vi "HEWH Flow Temp Adjust.vi"(0 "Core HEWH Data in":T5={"Scan Rate Adjust"=0.0, "Draw Count"=0, "Test Patten Setup"={"Total Gallons Schedule"=[], "PRAT/RLT Sequence"=[{"Sequence #"=1.0, "Cycles"=35, "Mode Setting"="", "Flow Rate (GPM)"=0.0, "Temperature (F)"=0.0, "Reset Timer"=FALSE, "Use Temp Decline Method"=FALSE, "Terminate Condition"=enum."C1-Terminate Draw @ Gallon Mark", "Condition Value #1"=0.0, "UE"=FALSE, "LE"=FALSE, "Comp"=FALSE, "Fan"=FALSE, "Test End Time (Sec)"=0.0, "Purge Until Cutout"=FALSE, "Start Conditions"=enum."Heat Source Cutout", "Condition Value #2"=0.0, "Remove Power"=FALSE, "Time"=0.0, "Check Special Cond."=enum."SC1-Do Nothing", "Condition#"=enum."C1", "Draw Flags"=enum."N/A", "Data Processing Delay (FHD 15sec, UEF 5 Sec)"=0.0, "Test Complete"=FALSE}, {"Sequence #"=2.0, "Cycles"=15, "Mode Setting"="", "Flow Rate (GPM)"=0.0, "Temperature (F)"=0.0, "Reset Timer"=FALSE, "Use Temp Decline Method"=FALSE, "Terminate Condition"=enum."C1-Terminate Draw @ Gallon Mark", "Condition Value #1"=0.0, "UE"=FALSE, "LE"=FALSE, "Comp"=FALSE, "Fan"=FALSE, "Test End Time (Sec)"=0.0, "Purge Until Cutout"=FALSE, "Start Conditions"=enum."Heat Source Cutout", "Condition Value #2"=0.0, "Remove Power"=FALSE, "Time"=0.0, "Check Special Cond."=enum."SC1-Do Nothing", "Condition#"=enum."C1", "Draw Flags"=enum."N/A", "Data Processing Delay (FHD 15sec, UEF 5 Sec)"=0.0, "Test Complete"=FALSE}, {"Sequence #"=3.0, "Cycles"=35, "Mode Setting"="", "Flow Rate (GPM)"=0.0, "Temperature (F)"=0.0, "Reset Timer"=FALSE, "Use Temp Decline Method"=FALSE, "Terminate Condition"=enum."C1-Terminate Draw @ Gallon Mark", "Condition Value #1"=0.0, "UE"=FALSE, "LE"=FALSE, "Comp"=FALSE, "Fan"=FALSE, "Test End Time (Sec)"=0.0, "Purge Until Cutout"=FALSE, "Start Conditions"=enum."Heat Source Cutout", "Condition Value #2"=0.0, "Remove Power"=FALSE, "Time"=0.0, "Check Special Cond."=enum."SC1-Do Nothing", "Condition#"=enum."C1", "Draw Flags"=enum."N/A", "Data Processing Delay (FHD 15sec, UEF 5 Sec)"=0.0, "Test Complete"=FALSE}, {"Sequence #"=4.0, "Cycles"=15, "Mode Setting"="", "Flow Rate (GPM)"=0.0, "Temperature (F)"=0.0, "Reset Timer"=FALSE, "Use Temp Decline Method"=FALSE, "Terminate Condition"=enum."C1-Terminate Draw @ Gallon Mark", "Condition Value #1"=0.0, "UE"=FALSE, "LE"=FALSE, "Comp"=FALSE, "Fan"=FALSE, "Test End Time (Sec)"=0.0, "Purge Until Cutout"=FALSE, "Start Conditions"=enum."Heat Source Cutout", "Condition Value #2"=0.0, "Remove Power"=FALSE, "Time"=0.0, "Check Special Cond."=enum."SC1-Do Nothing", "Condition#"=enum."C1", "Draw Flags"=enum."N/A", "Data Processing Delay (FHD 15sec, UEF 5 Sec)"=0.0, "Test Complete"=FALSE}, {"Sequence #"=5.0, "Cycles"=35, "Mode Setting"="", "Flow Rate (GPM)"=0.0, "Temperature (F)"=0.0, "Reset Timer"=FALSE, "Use Temp Decline Method"=FALSE, "Terminate Condition"=enum."C1-Terminate Draw @ Gallon Mark", "Condition Value #1"=0.0, "UE"=FALSE, "LE"=FALSE, "Comp"=FALSE, "Fan"=FALSE, "Test End Time (Sec)"=0.0, "Purge Until Cutout"=FALSE, "Start Conditions"=enum."Heat Source Cutout", "Condition Value #2"=0.0, "Remove Power"=FALSE, "Time"=0.0, "Check Special Cond."=enum."SC1-Do Nothing", "Condition#"=enum."C1", "Draw Flags"=enum."N/A", "Data Processing Delay (FHD 15sec, UEF 5 Sec)"=0.0, "Test Complete"=FALSE}, {"Sequence #"=6.0, "Cycles"=15, "Mode Setting"="", "Flow Rate (GPM)"=0.0, "Temperature (F)"=0.0, "Reset Timer"=FALSE, "Use Temp Decline Method"=FALSE, "Terminate Condition"=enum."C1-Terminate Draw @ Gallon Mark", "Condition Value #1"=0.0, "UE"=FALSE, "LE"=FALSE, "Comp"=FALSE, "Fan"=FALSE, "Test End Time (Sec)"=0.0, "Purge Until Cutout"=FALSE, "Start Conditions"=enum."Heat Source Cutout", "Condition Value #2"=0.0, "Remove Power"=FALSE, "Time"=0.0, "Check Special Cond."=enum."SC1-Do Nothing", "Condition#"=enum."C1", "Draw Flags"=enum."N/A", "Data Processing Delay (FHD 15sec, UEF 5 Sec)"=0.0, "Test Complete"=FALSE}, {"Sequence #"=7.0, "Cycles"=35, "Mode Setting"="", "Flow Rate (GPM)"=0.0, "Temperature (F)"=0.0, "Reset Timer"=FALSE, "Use Temp Decline Method"=FALSE, "Terminate Condition"=enum."C1-Terminate Draw @ Gallon Mark", "Condition Value #1"=0.0, "UE"=FALSE, "LE"=FALSE, "Comp"=FALSE, "Fan"=FALSE, "Test End Time (Sec)"=0.0, "Purge Until Cutout"=FALSE, "Start Conditions"=enum."Heat Source Cutout", "Condition Value #2"=0.0, "Remove Power"=FALSE, "Time"=0.0, "Check Special Cond."=enum."SC1-Do Nothing", "Condition#"=enum."C1", "Draw Flags"=enum."N/A", "Data Processing Delay (FHD 15sec, UEF 5 Sec)"=0.0, "Test Complete"=FALSE}, {"Sequence #"=8.0, "Cycles"=15, "Mode Setting"="", "Flow Rate (GPM)"=0.0, "Temperature (F)"=0.0, "Reset Timer"=FALSE, "Use Temp Decline Method"=FALSE, "Terminate Condition"=enum."C1-Terminate Draw @ Gallon Mark", "Condition Value #1"=0.0, "UE"=FALSE, "LE"=FALSE, "Comp"=FALSE, "Fan"=FALSE, "Test End Time (Sec)"=0.0, "Purge Until Cutout"=FALSE, "Start Conditions"=enum."Heat Source Cutout", "Condition Value #2"=0.0, "Remove Power"=FALSE, "Time"=0.0, "Check Special Cond."=enum."SC1-Do Nothing", "Condition#"=enum."C1", "Draw Flags"=enum."N/A", "Data Processing Delay (FHD 15sec, UEF 5 Sec)"=0.0, "Test Complete"=FALSE}], "Current Sequence Index"=0}, "HEWH Specific DAQ"={"HEWH Data"={"HEWH Standard"={"Voltage (Volts)"=0.0, "Current (Amps)"=0.0, "Power (Watts)"=0.0, "WattHours (Wh)"=0.0, "TC Tree (AVG)"=0.0, "Flow Rate (GPM)"=0.0, "Gallons (Gal)"=0.0, "RTD Out (Deg F)"=0.0, "RTD In (Deg F)"=0.0, "RTD Amb (Deg F)"=0.0, "TC Down"=0.0, "UE Event Lead"=0, "LE Event Lead"=0, "TC Tree Array"=[]}, "PRAT"={"Power (Watts) A"=4192.0, "Power (Watts) B"=4192.0, "Power (Watts) C"=4192.0, "Power (Watts) D"=4192.0, "TC1"=0.0, "TC2"=0.0, "TC3"=0.0, "TC4"=0.0, "WattHours (Wh) A"=4192.0, "WattHours (Wh) B"=4192.0, "WattHours (Wh) C"=4192.0, "WattHours (Wh) D"=4192.0, "Ambient"=0.0, "Extra Temp"=0.0}, "Additional Power Data"={"Vthd"=236.2, "Frequency (Hz)"=236.2, "Apparent Power (VA)"=236.2, "Power Factor"=236.2, "Current Crest Factor"=236.2, "Voltage Crest Factor"=236.2, "Integration Time (sec)"=236.2}}, "Flow Valve % Open"=0.0, "Power State"={"UE"=FALSE, "LE"=FALSE, "COMP"=FALSE, "FANS"=FALSE}, "Power Analyzer"=enum."", "Flow Valve uA Output"=0, "Gallons Start (Gal)"=0.0}, "Test Output Data"={"PreDraw Data Table"=[], "Data Table"=[], "MW100 TC Headers"=[]}, "Calc and Calibration"={"Mean SD Var Max Min Array"=[], "Draw Statistics (DBL)"=[], "Calibration Coefficients DBL"=[], "Start Gallons"=0.0, "Starting Temp Decline"=0.0, "K-Factor (Intellifaucet)"=0.0, "All Draw Stats"=[], "RTD Terminate Value"=0.0}, "Current Draw Time"=0.0, "LV Program"=enum."HEWH", "Station ID"=enum."A", "Current Cond"=enum."N/A", "Test Complete"=FALSE} {"Test Patten Setup"."PRAT/RLT Sequence"."Time" format="%<%H:%M:%S>t"; "Test Patten Setup"."Total Gallons Schedule" format="%.2f"}, 1 "MW100":refnum<visa-resource-name>, 2 "Yokogawa WT210":refnum<visa-resource-name>, 3 "Temperature":T2 format="%.2f", 4 "Gallon Target":T2=10.72 format="%.2f", 5 "error in (no error)":errorcluster, 6 "Debug":bool, 7 "Purge Time (Seconds)":T2=180.0 format="%.2f", 8 "Use Fuzzy Logic":bool, 9 "PID gains (Temp)":T1={"proportional gain (Kc)"=0.1, "integral time (Ti, min)"=0.01, "derivative time (Td, min)"=0.0} {"derivative time (Td, min)" format="%.3f"; "integral time (Ti, min)" format="%.3f"; "proportional gain (Kc)" format="%.3f"}, 10 "GEA2?":bool, 11 "GPM Target":T2=3.0 format="%.2f", 12 "State":T4, 13 "MW100 Sema":T3, 16 "Use Emerson 5700?":bool, 17 "Pressurization Time (sec)":i32, 18 "Laurel IP Address":string) -> (14 "Core HEWH Data out":T5={"Scan Rate Adjust"=0.0, "Draw Count"=0, "Test Patten Setup"={"Total Gallons Schedule"=[], "PRAT/RLT Sequence"=[{"Sequence #"=1.0, "Cycles"=35, "Mode Setting"="", "Flow Rate (GPM)"=0.0, "Temperature (F)"=0.0, "Reset Timer"=FALSE, "Use Temp Decline Method"=FALSE, "Terminate Condition"=enum."C1-Terminate Draw @ Gallon Mark", "Condition Value #1"=0.0, "UE"=FALSE, "LE"=FALSE, "Comp"=FALSE, "Fan"=FALSE, "Test End Time (Sec)"=0.0, "Purge Until Cutout"=FALSE, "Start Conditions"=enum."Heat Source Cutout", "Condition Value #2"=0.0, "Remove Power"=FALSE, "Time"=0.0, "Check Special Cond."=enum."SC1-Do Nothing", "Condition#"=enum."C1", "Draw Flags"=enum."N/A", "Data Processing Delay (FHD 15sec, UEF 5 Sec)"=0.0, "Test Complete"=FALSE}, {"Sequence #"=2.0, "Cycles"=15, "Mode Setting"="", "Flow Rate (GPM)"=0.0, "Temperature (F)"=0.0, "Reset Timer"=FALSE, "Use Temp Decline Method"=FALSE, "Terminate Condition"=enum."C1-Terminate Draw @ Gallon Mark", "Condition Value #1"=0.0, "UE"=FALSE, "LE"=FALSE, "Comp"=FALSE, "Fan"=FALSE, "Test End Time (Sec)"=0.0, "Purge Until Cutout"=FALSE, "Start Conditions"=enum."Heat Source Cutout", "Condition Value #2"=0.0, "Remove Power"=FALSE, "Time"=0.0, "Check Special Cond."=enum."SC1-Do Nothing", "Condition#"=enum."C1", "Draw Flags"=enum."N/A", "Data Processing Delay (FHD 15sec, UEF 5 Sec)"=0.0, "Test Complete"=FALSE}, {"Sequence #"=3.0, "Cycles"=35, "Mode Setting"="", "Flow Rate (GPM)"=0.0, "Temperature (F)"=0.0, "Reset Timer"=FALSE, "Use Temp Decline Method"=FALSE, "Terminate Condition"=enum."C1-Terminate Draw @ Gallon Mark", "Condition Value #1"=0.0, "UE"=FALSE, "LE"=FALSE, "Comp"=FALSE, "Fan"=FALSE, "Test End Time (Sec)"=0.0, "Purge Until Cutout"=FALSE, "Start Conditions"=enum."Heat Source Cutout", "Condition Value #2"=0.0, "Remove Power"=FALSE, "Time"=0.0, "Check Special Cond."=enum."SC1-Do Nothing", "Condition#"=enum."C1", "Draw Flags"=enum."N/A", "Data Processing Delay (FHD 15sec, UEF 5 Sec)"=0.0, "Test Complete"=FALSE}, {"Sequence #"=4.0, "Cycles"=15, "Mode Setting"="", "Flow Rate (GPM)"=0.0, "Temperature (F)"=0.0, "Reset Timer"=FALSE, "Use Temp Decline Method"=FALSE, "Terminate Condition"=enum."C1-Terminate Draw @ Gallon Mark", "Condition Value #1"=0.0, "UE"=FALSE, "LE"=FALSE, "Comp"=FALSE, "Fan"=FALSE, "Test End Time (Sec)"=0.0, "Purge Until Cutout"=FALSE, "Start Conditions"=enum."Heat Source Cutout", "Condition Value #2"=0.0, "Remove Power"=FALSE, "Time"=0.0, "Check Special Cond."=enum."SC1-Do Nothing", "Condition#"=enum."C1", "Draw Flags"=enum."N/A", "Data Processing Delay (FHD 15sec, UEF 5 Sec)"=0.0, "Test Complete"=FALSE}, {"Sequence #"=5.0, "Cycles"=35, "Mode Setting"="", "Flow Rate (GPM)"=0.0, "Temperature (F)"=0.0, "Reset Timer"=FALSE, "Use Temp Decline Method"=FALSE, "Terminate Condition"=enum."C1-Terminate Draw @ Gallon Mark", "Condition Value #1"=0.0, "UE"=FALSE, "LE"=FALSE, "Comp"=FALSE, "Fan"=FALSE, "Test End Time (Sec)"=0.0, "Purge Until Cutout"=FALSE, "Start Conditions"=enum."Heat Source Cutout", "Condition Value #2"=0.0, "Remove Power"=FALSE, "Time"=0.0, "Check Special Cond."=enum."SC1-Do Nothing", "Condition#"=enum."C1", "Draw Flags"=enum."N/A", "Data Processing Delay (FHD 15sec, UEF 5 Sec)"=0.0, "Test Complete"=FALSE}, {"Sequence #"=6.0, "Cycles"=15, "Mode Setting"="", "Flow Rate (GPM)"=0.0, "Temperature (F)"=0.0, "Reset Timer"=FALSE, "Use Temp Decline Method"=FALSE, "Terminate Condition"=enum."C1-Terminate Draw @ Gallon Mark", "Condition Value #1"=0.0, "UE"=FALSE, "LE"=FALSE, "Comp"=FALSE, "Fan"=FALSE, "Test End Time (Sec)"=0.0, "Purge Until Cutout"=FALSE, "Start Conditions"=enum."Heat Source Cutout", "Condition Value #2"=0.0, "Remove Power"=FALSE, "Time"=0.0, "Check Special Cond."=enum."SC1-Do Nothing", "Condition#"=enum."C1", "Draw Flags"=enum."N/A", "Data Processing Delay (FHD 15sec, UEF 5 Sec)"=0.0, "Test Complete"=FALSE}, {"Sequence #"=7.0, "Cycles"=35, "Mode Setting"="", "Flow Rate (GPM)"=0.0, "Temperature (F)"=0.0, "Reset Timer"=FALSE, "Use Temp Decline Method"=FALSE, "Terminate Condition"=enum."C1-Terminate Draw @ Gallon Mark", "Condition Value #1"=0.0, "UE"=FALSE, "LE"=FALSE, "Comp"=FALSE, "Fan"=FALSE, "Test End Time (Sec)"=0.0, "Purge Until Cutout"=FALSE, "Start Conditions"=enum."Heat Source Cutout", "Condition Value #2"=0.0, "Remove Power"=FALSE, "Time"=0.0, "Check Special Cond."=enum."SC1-Do Nothing", "Condition#"=enum."C1", "Draw Flags"=enum."N/A", "Data Processing Delay (FHD 15sec, UEF 5 Sec)"=0.0, "Test Complete"=FALSE}, {"Sequence #"=8.0, "Cycles"=15, "Mode Setting"="", "Flow Rate (GPM)"=0.0, "Temperature (F)"=0.0, "Reset Timer"=FALSE, "Use Temp Decline Method"=FALSE, "Terminate Condition"=enum."C1-Terminate Draw @ Gallon Mark", "Condition Value #1"=0.0, "UE"=FALSE, "LE"=FALSE, "Comp"=FALSE, "Fan"=FALSE, "Test End Time (Sec)"=0.0, "Purge Until Cutout"=FALSE, "Start Conditions"=enum."Heat Source Cutout", "Condition Value #2"=0.0, "Remove Power"=FALSE, "Time"=0.0, "Check Special Cond."=enum."SC1-Do Nothing", "Condition#"=enum."C1", "Draw Flags"=enum."N/A", "Data Processing Delay (FHD 15sec, UEF 5 Sec)"=0.0, "Test Complete"=FALSE}], "Current Sequence Index"=0}, "HEWH Specific DAQ"={"HEWH Data"={"HEWH Standard"={"Voltage (Volts)"=0.0, "Current (Amps)"=0.0, "Power (Watts)"=0.0, "WattHours (Wh)"=0.0, "TC Tree (AVG)"=0.0, "Flow Rate (GPM)"=0.0, "Gallons (Gal)"=0.0, "RTD Out (Deg F)"=0.0, "RTD In (Deg F)"=0.0, "RTD Amb (Deg F)"=0.0, "TC Down"=0.0, "UE Event Lead"=0, "LE Event Lead"=0, "TC Tree Array"=[]}, "PRAT"={"Power (Watts) A"=4192.0, "Power (Watts) B"=4192.0, "Power (Watts) C"=4192.0, "Power (Watts) D"=4192.0, "TC1"=0.0, "TC2"=0.0, "TC3"=0.0, "TC4"=0.0, "WattHours (Wh) A"=4192.0, "WattHours (Wh) B"=4192.0, "WattHours (Wh) C"=4192.0, "WattHours (Wh) D"=4192.0, "Ambient"=0.0, "Extra Temp"=0.0}, "Additional Power Data"={"Vthd"=236.2, "Frequency (Hz)"=236.2, "Apparent Power (VA)"=236.2, "Power Factor"=236.2, "Current Crest Factor"=236.2, "Voltage Crest Factor"=236.2, "Integration Time (sec)"=236.2}}, "Flow Valve % Open"=0.0, "Power State"={"UE"=FALSE, "LE"=FALSE, "COMP"=FALSE, "FANS"=FALSE}, "Power Analyzer"=enum."", "Flow Valve uA Output"=0, "Gallons Start (Gal)"=0.0}, "Test Output Data"={"PreDraw Data Table"=[], "Data Table"=[], "MW100 TC Headers"=[]}, "Calc and Calibration"={"Mean SD Var Max Min Array"=[], "Draw Statistics (DBL)"=[], "Calibration Coefficients DBL"=[], "Start Gallons"=0.0, "Starting Temp Decline"=0.0, "K-Factor (Intellifaucet)"=0.0, "All Draw Stats"=[], "RTD Terminate Value"=0.0}, "Current Draw Time"=0.0, "LV Program"=enum."HEWH", "Station ID"=enum."A", "Current Cond"=enum."N/A", "Test Complete"=FALSE} {"Test Patten Setup"."PRAT/RLT Sequence"."Time" format="%<%H:%M:%S>t"; "Test Patten Setup"."Total Gallons Schedule" format="%.2f"}, 15 "MW100 Out":refnum<visa-resource-name>, 19 "error out":errorcluster)   [LabVIEW 2016]
uses:
  Utility/Custom Pallet Controls/Custom Pallet DBL.ctl
  Type Definitions/HEWH Output Information.ctl
  Type Definitions/HEWH Draw Pattern Setup.ctl
  Type Definitions/PRAT Test.ctl
  Utility/Save File/File Setup (Public)/Type Definition/Save File HEWH Heating Control Mode.ctl
  Type Definitions/Terminate Draw Conditions.ctl
  Type Definitions/HEWH Start Conditions.ctl
  Type Definitions/Check Special Condtions.ctl
  Type Definitions/HEWH Special Condition Check.ctl
  Type Definitions/HEWH Draw Flag ENUM.ctl
  Type Definitions/HEWH Specific DAQ.ctl
  Type Definitions/HEWH Power Data.ctl
  Type Definitions/HEWH Power Elements.ctl
  Utility/Type Definitions/UTILITY Power Analyzer.ctl
  Type Definitions/HEWH Calc and Calibration.ctl
  Utility/Save File/File Setup (Public)/Type Definition/Save File DOE LabView Program.ctl
  Custom Instrument Control/MW100/Type Definitions/Station ID Selector.ctl
  Type Definitions/HEWH Purge Draw.ctl
  <vilib>/ptbypt/NI_PtbyPt.lvlib
  Utility/Save File/File Setup.lvlib
panel:
  out "Adjusting Temp":bool
  in  "Adjust Temp Timer":dbl=0.5 format="%#_13g"
  out "Elapsed Time (sec)":dbl
  out "Time to Draw Water (Seconds)":T2 format="%.2f"
  out "Loop Rate":dbl format="%0.2f"
  out "Gallons":dbl(graph)
  out "Intellifaucet %Open":dbl(graph)
  out "GPM":dbl(graph)
  out "TC Down":dbl(graph)
  # "Draw Pattern Setup (24 Hour)"
  # "Draw Pattern Setup (24 Hour)"
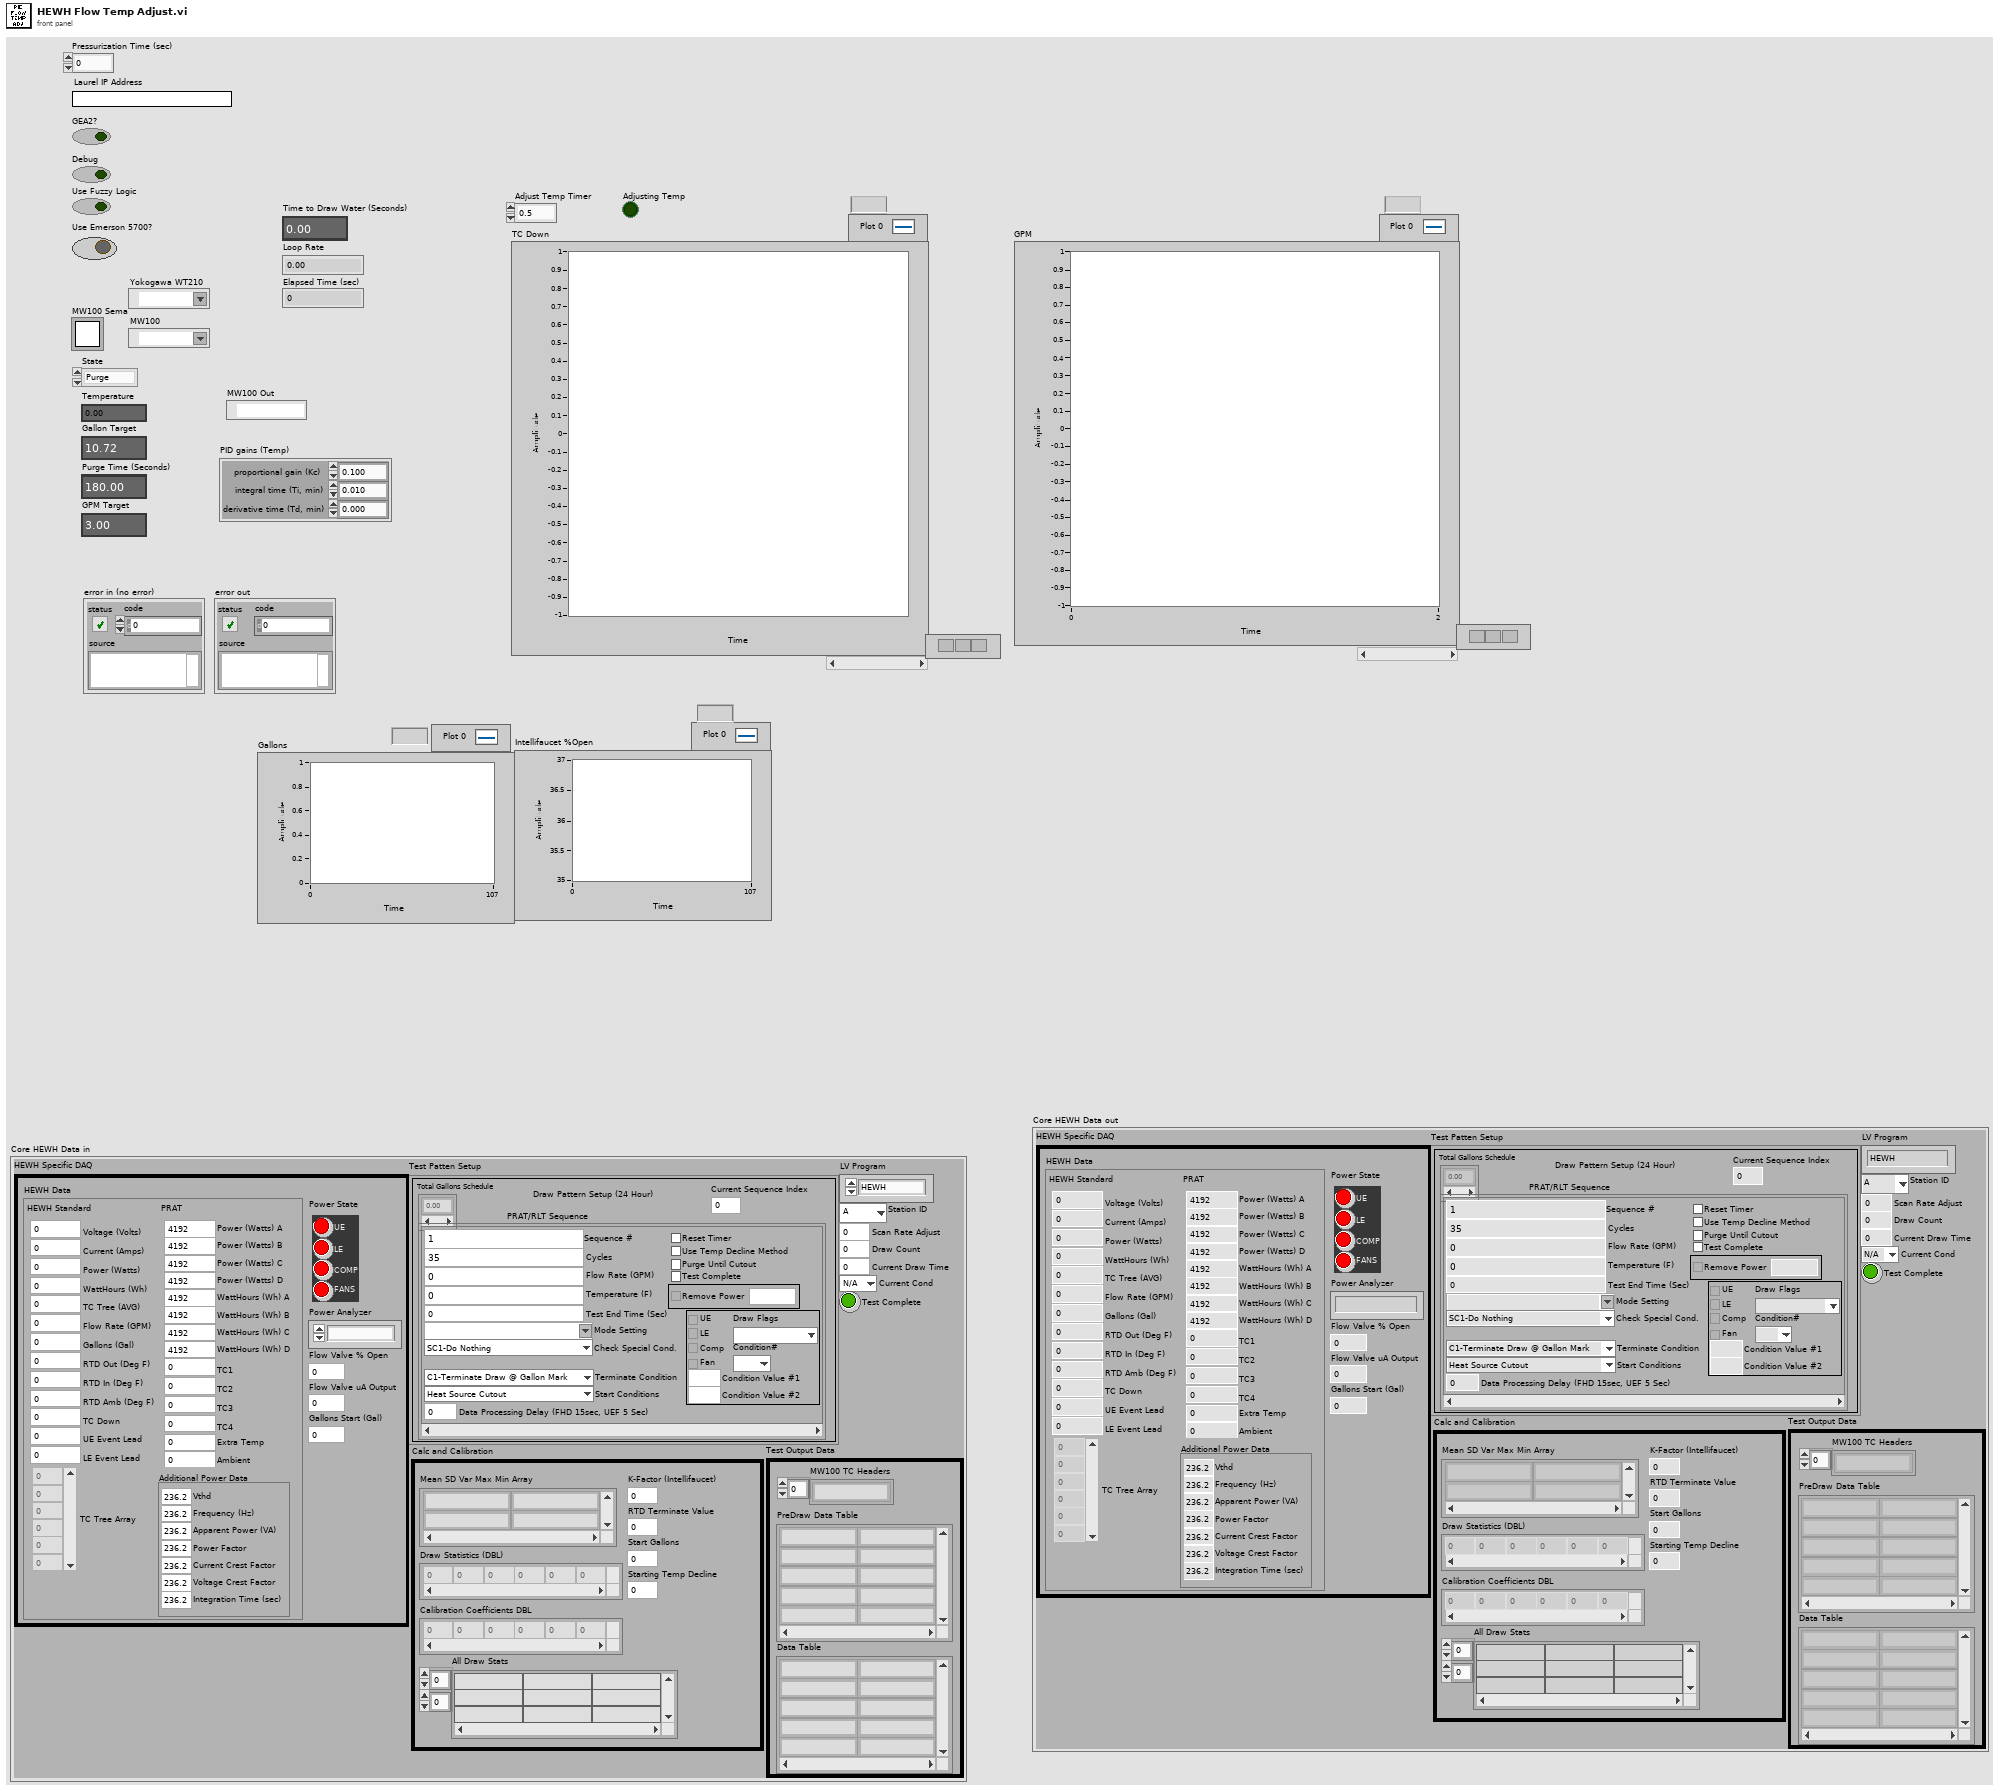
[diagram p1: front panel]
types:
  T1 = cluster{"proportional gain (Kc)":dbl, "integral time (Ti, min)":dbl, "derivative time (Td, min)":dbl}
  T2 = typedef "Custom Pallet DBL.ctl" = dbl
  T3 = typedef "Semaphore RefNum" = refnum<k1>
  T4 = typedef "HEWH Purge Draw.ctl" = enum16{"Purge", "Draw"}
  T5 = typedef "HEWH Output Information.ctl" = cluster{"Scan Rate Adjust":dbl, "Draw Count":i32, "Test Patten Setup":T6, "HEWH Specific DAQ":T14, "Test Output Data":cluster{"PreDraw Data Table":string[][], "Data Table":string[][], "MW100 TC Headers":string[]}, "Calc and Calibration":T18, "Current Draw Time":dbl, "LV Program":T19, "Station ID":T20, "Current Cond":T12, "Test Complete":bool}
  T6 = typedef "HEWH Draw Pattern Setup.ctl" = cluster{"Total Gallons Schedule":dbl[], "PRAT/RLT Sequence":T7[], "Current Sequence Index":i32}
  T7 = typedef "PRAT Test.ctl" = cluster{"Sequence #":dbl, "Cycles":i32, "Mode Setting":T8, "Flow Rate (GPM)":dbl, "Temperature (F)":dbl, "Reset Timer":bool, "Use Temp Decline Method":bool, "Terminate Condition":T9, "Condition Value #1":dbl, "UE":bool, "LE":bool, "Comp":bool, "Fan":bool, "Test End Time (Sec)":dbl, "Purge Until Cutout":bool, "Start Conditions":T10, "Condition Value #2":dbl, "Remove Power":bool, "Time":dbl, "Check Special Cond.":T11, "Condition#":T12, "Draw Flags":T13, "Data Processing Delay (FHD 15sec, UEF 5 Sec)":dbl, "Test Complete":bool}
  T8 = typedef "File Setup.lvlib/Save File HEWH Heating Control Mode.ctl" = string
  T9 = typedef "Terminate Draw Conditions.ctl" = enum16{"C1-Terminate Draw @ Gallon Mark", "C2-Special Last Draw (HU Test)", "C3-RTD Out <=", "C4-Mean Tank Temp <=", "C5-Decrease RTD Out (Deg F)", "C6-Time (Seconds)", "C7-Until Any Heat Source", "C8-Specific Heat Source", "C9-Do Nothing"}
  T10 = typedef "HEWH Start Conditions.ctl" = enum16{"Heat Source Cutout", "At Time (Seconds)", "Every X (Seconds)", "T2 >= X° Below Setpoint", "Seconds From Complete", "Wait for LE & Comp Cutout", "Wait for Comp Cutout", "Wait for LE Cutout", "Wait for UE Cutout"}
  T11 = typedef "Check Special Condtions.ctl" = enum16{"SC1-Do Nothing", "SC2-Check Heat Source (On-C2/Off-C1)", "SC3-Check Skip Condition", "SC4-Check Heat Source ON/Fail"}
  T12 = typedef "HEWH Special Condition Check.ctl" = enum16{"N/A", "C1", "C2", "Reset/Fail", "Skip Draw Sequence"}
  T13 = typedef "HEWH Draw Flag ENUM.ctl" = enum16{"N/A", "None(0)", "Sml(1)", "Med(2)", "SmlMed(3)", "Lrg(4)", "SmlLrg(5)", "MedLrg(6)", "SmlMedLrg(7)"}
  T14 = typedef "HEWH Specific DAQ.ctl" = cluster{"HEWH Data":T15, "Flow Valve % Open":dbl, "Power State":T16, "Power Analyzer":T17, "Flow Valve uA Output":i32, "Gallons Start (Gal)":dbl}
  T15 = typedef "HEWH Power Data.ctl" = cluster{"HEWH Standard":cluster{"Voltage (Volts)":dbl, "Current (Amps)":dbl, "Power (Watts)":dbl, "WattHours (Wh)":dbl, "TC Tree (AVG)":dbl, "Flow Rate (GPM)":dbl, "Gallons (Gal)":dbl, "RTD Out (Deg F)":dbl, "RTD In (Deg F)":dbl, "RTD Amb (Deg F)":dbl, "TC Down":dbl, "UE Event Lead":i32, "LE Event Lead":i32, "TC Tree Array":dbl[]}, "PRAT":cluster{"Power (Watts) A":dbl, "Power (Watts) B":dbl, "Power (Watts) C":dbl, "Power (Watts) D":dbl, "TC1":dbl, "TC2":dbl, "TC3":dbl, "TC4":dbl, "WattHours (Wh) A":dbl, "WattHours (Wh) B":dbl, "WattHours (Wh) C":dbl, "WattHours (Wh) D":dbl, "Ambient":dbl, "Extra Temp":dbl}, "Additional Power Data":cluster{"Vthd":dbl, "Frequency (Hz)":dbl, "Apparent Power (VA)":dbl, "Power Factor":dbl, "Current Crest Factor":dbl, "Voltage Crest Factor":dbl, "Integration Time (sec)":dbl}}
  T16 = typedef "HEWH Power Elements.ctl" = cluster{"UE":bool, "LE":bool, "COMP":bool, "FANS":bool}
  T17 = typedef "UTILITY Power Analyzer.ctl" = enum16{"", "APLUS", "WT210", "WT500", "WT300", "OSI", "Debug", "WT230", "WT300_1", "WT300_2"}
  T18 = typedef "HEWH Calc and Calibration.ctl" = cluster{"Mean SD Var Max Min Array":string[][], "Draw Statistics (DBL)":dbl[][], "Calibration Coefficients DBL":dbl[][], "Start Gallons":dbl, "Starting Temp Decline":dbl, "K-Factor (Intellifaucet)":dbl, "All Draw Stats":string[][], "RTD Terminate Value":dbl}
  T19 = typedef "File Setup.lvlib/Save File DOE LabView Program.ctl" = enum16{"No Name Found", "DOE Stand", "Dishwasher Kitchen", "Portable Stand", "HEWH", "Dryer", "Dryer WILT", "HCC", "PRAT", "HEWH RLT", "Refrigeration"}
  T20 = typedef "Station ID Selector.ctl" = enum16{"", "A", "B", "C", "D", "Global"}
  T21 = typedef "Emerson 5700 Data.ctl" = cluster{"Mass Flow Rate (Scaled Integer)":u16, "Density (Scaled Integer)":u16, "Temperature (Scaled Integer)":u16, "Volume Flow Rate (Scaled Integer)":u16, "Totalizer 1 (Scaled Integer)":u16, "Totalizer 2 (Scaled Integer)":u16, "Transmitter Software Rev":u16, "Flow Direction":string, "Mass Flow Units":string, "Density Units":string, "Temperature Units":string, "Volume Flow Units":string, "Pressure Units":string, "Mass Total Units":string, "Volume Total Units":string, "Inventory 1 (Scaled Integer)":u16, "Inventory 2 (Scaled Integer)":u16, "Mass Flow Rate":dbl, "Density":dbl, "Temperature":dbl, "Volume Flow Rate":dbl, "Pressure (Scaled Integer)":u16, "Current Value Totalizer 1 (Pounds per draw)":dbl, "Current Value Totalizer 2 (Gallons per draw)":dbl, "Current Value Inventory 1 (Pounds Total)":dbl, "Current Value Inventory 2 (Gallons Total)":dbl, "Drive Gain":dbl, "Raw Tube Frequency (Hz)":dbl, "Dynamic Viscosity (Centipoise)":dbl, "Kinematic Viscosity (Centistokes)":dbl, "Hot Gallons (Calculated Gallons)":dbl, "Hot Flow Rate (Calculated GPM)":dbl, "Hot Gallons Inventory (Gallons)":dbl}
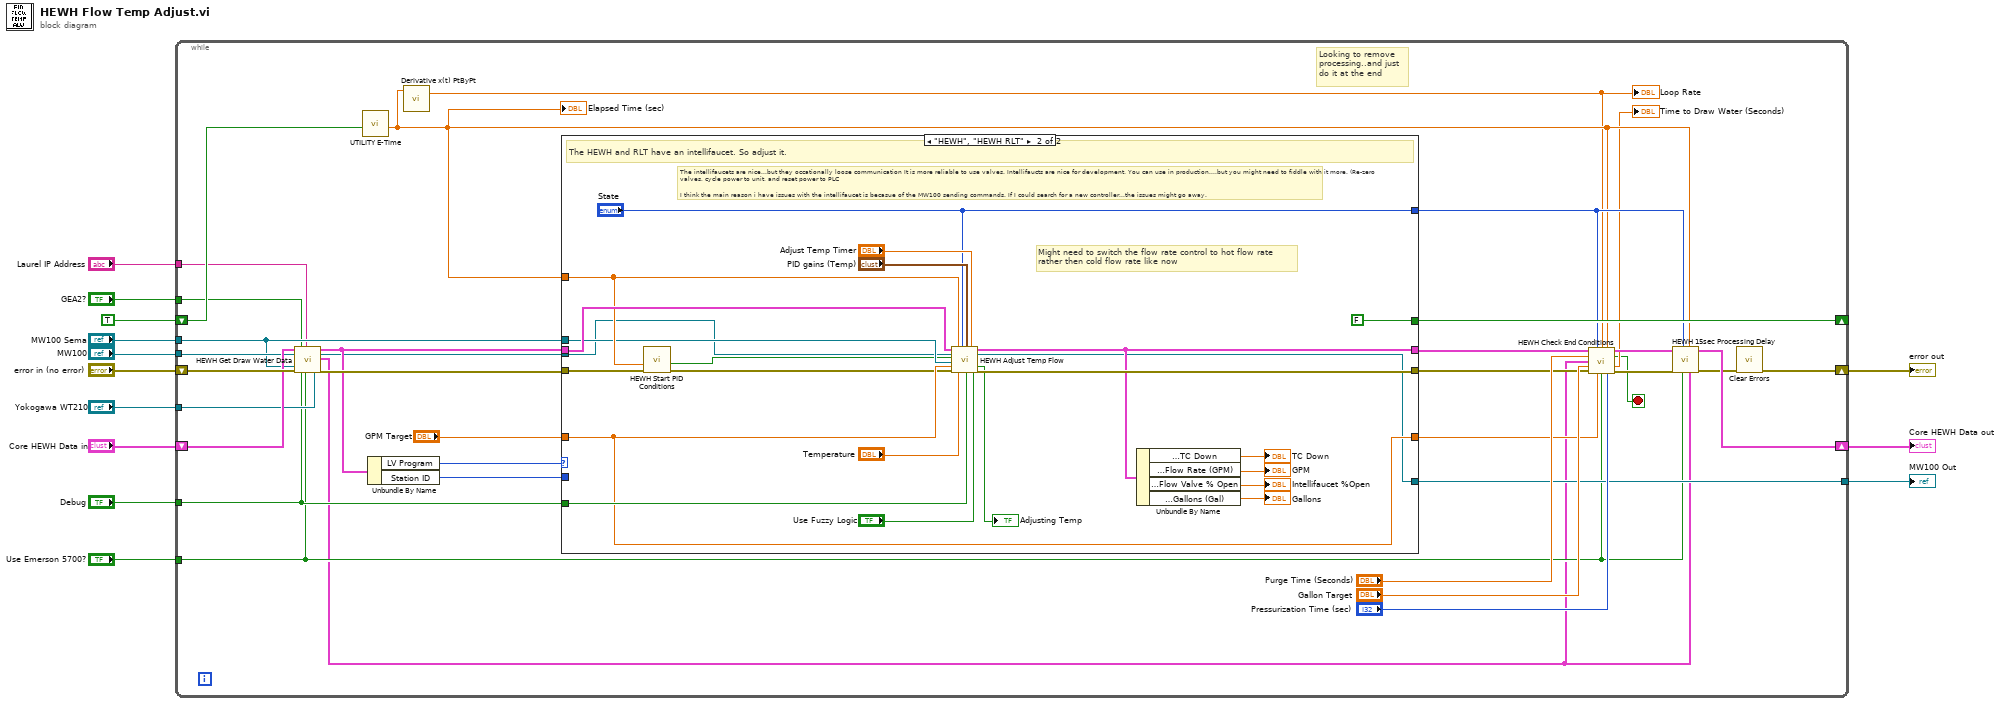
[diagram p0: block diagram]
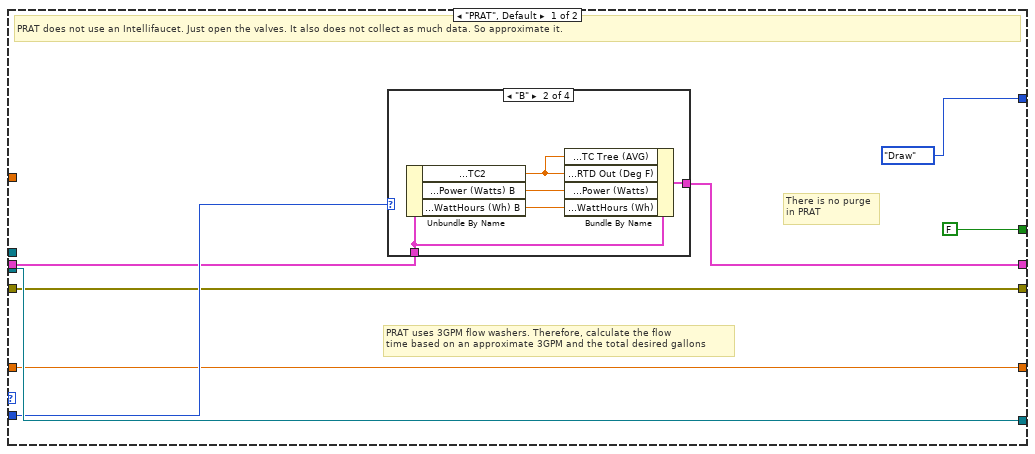
[diagram p2: hidden frame]
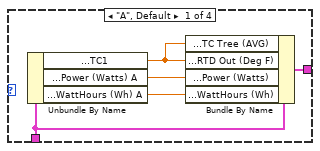
[diagram p3: hidden frame]
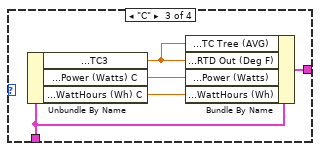
[diagram p4: hidden frame]
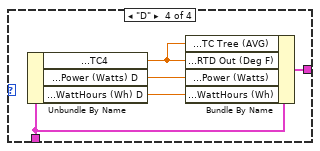
[diagram p5: hidden frame]
diagram:
  n1 = while {
    shift-right: [w42] -> w11
    shift-left: "Core HEWH Data in" -> [w38]
    shift-right: [w43] -> w10
    shift-left: "error in (no error)" -> [w40]
    tunnel: "MW100" -> [w36]
    tunnel: [w22] -> w13
    tunnel: "MW100 Sema" -> [w19]
    shift-right: [w45] -> _
    shift-left: TRUE ("Reset") -> [w46]
    tunnel: "Yokogawa WT210" -> [w21]
    tunnel: "Laurel IP Address" -> [w17]
    tunnel: "GEA2?" -> [w18]
    tunnel: "Debug" -> [w20]
    tunnel: "Use Emerson 5700?" -> [w15]
    stop <- w26 stop-if-true
    # "Looking to remove\nprocessing..and just\ndo it at the end"
    n2 = call "HEWH Get Draw Water Data.vi"("Core HEWH Data Input"=w38, "MW100 Input"=w36, "MW100 Sema in"=w19, "error in (no error)"=w40, "GEA2?"=w18, "Debug in"=w20, "Laurel IP Address"=w17, "Use Emerson 5700?"=w15, "Yokogawa WT210"=w21) -> ("Core HEWH Data Station A"=w37:T5, "MW100 Output"=w35:refnum<visa-resource-name>, "Emerson Flow Meter Data Output"=w14:T21, "error out"=w39:errorcluster)  [unwired: 7 in]
    n3 = call "UTILITY E-Time.vi"("Reset"=w46) -> ("Elapsed Time (sec)"=w31:dbl)  [unwired: 8 in, 2 out]
    "Elapsed Time (sec)" <- w31
    n4 = Unbundle By Name(w37) -> ("LV Program"=w48:T19, "Station ID"=w44:T20)
    n5 = call <vilib>:"Derivative x(t) PtByPt.vi"("x"=w31) -> ("dx/dt"=w24:dbl)  [unwired: 3 in, 1 out]
    "Loop Rate" <- w24
    n6 = case shown="\"HEWH\", \"HEWH RLT\"" w48 {
      tunnel: [w50 w94] -> w23
      tunnel: [w56 w89] -> w22
      tunnel: w35 -> [w56 w84]
      tunnel: w39 -> [w50 w87]
      tunnel: w37 -> [w51 w91]
      tunnel: [w52 w90] -> w16
      tunnel: w19 -> [_ w85]
      tunnel: w31 -> [_ w88]
      tunnel: "GPM Target" -> [w49 w92]
      tunnel: [FALSE ("Reset") FALSE ("Reset")] -> w45
      tunnel: w44 -> [w53 _]
      tunnel: [HEWH_Purge_Draw."Draw" ("State") "State"] -> w32
      tunnel: w20 -> [_ w93]
      tunnel: [w49 w92] -> w27
      frame "PRAT", Default {
        # "There is no purge\nin PRAT"
        # "PRAT uses 3GPM flow washers. Therefore, calculate the flow\ntime based on an approximate 3GPM and the total desired gallons"
        # "PRAT does not use an Intellifaucet. Just open the valves. It also does not collect as much data. So approximate it."
        n7 = case shown="\"B\"" w53 {
          tunnel: [w61 w64 w69 w74] -> w52
          tunnel: w51 -> [w60 w63 w68 w73]
          frame "A", Default {
            n8 = Unbundle By Name(w60) -> ("HEWH Specific DAQ.HEWH Data.PRAT.TC1"=w57:dbl, "HEWH Specific DAQ.HEWH Data.PRAT.Power (Watts) A"=w59:dbl, "HEWH Specific DAQ.HEWH Data.PRAT.WattHours (Wh) A"=w58:dbl)
            n9 = Bundle By Name(cluster=w60, "HEWH Specific DAQ.HEWH Data.HEWH Standard.TC Tree (AVG)"=w57, "HEWH Specific DAQ.HEWH Data.HEWH Standard.RTD Out (Deg F)"=w57, "HEWH Specific DAQ.HEWH Data.HEWH Standard.Power (Watts)"=w59, "HEWH Specific DAQ.HEWH Data.HEWH Standard.WattHours (Wh)"=w58) -> (w61:T5)
          }
          frame "B" {
            n10 = Unbundle By Name(w63) -> ("HEWH Specific DAQ.HEWH Data.PRAT.TC2"=w62:dbl, "HEWH Specific DAQ.HEWH Data.PRAT.Power (Watts) B"=w66:dbl, "HEWH Specific DAQ.HEWH Data.PRAT.WattHours (Wh) B"=w65:dbl)
            n11 = Bundle By Name(cluster=w63, "HEWH Specific DAQ.HEWH Data.HEWH Standard.TC Tree (AVG)"=w62, "HEWH Specific DAQ.HEWH Data.HEWH Standard.RTD Out (Deg F)"=w62, "HEWH Specific DAQ.HEWH Data.HEWH Standard.Power (Watts)"=w66, "HEWH Specific DAQ.HEWH Data.HEWH Standard.WattHours (Wh)"=w65) -> (w64:T5)
          }
          frame "C" {
            n12 = Unbundle By Name(w68) -> ("HEWH Specific DAQ.HEWH Data.PRAT.TC3"=w67:dbl, "HEWH Specific DAQ.HEWH Data.PRAT.Power (Watts) C"=w70:dbl, "HEWH Specific DAQ.HEWH Data.PRAT.WattHours (Wh) C"=w71:dbl)
            n13 = Bundle By Name(cluster=w68, "HEWH Specific DAQ.HEWH Data.HEWH Standard.TC Tree (AVG)"=w67, "HEWH Specific DAQ.HEWH Data.HEWH Standard.RTD Out (Deg F)"=w67, "HEWH Specific DAQ.HEWH Data.HEWH Standard.Power (Watts)"=w70, "HEWH Specific DAQ.HEWH Data.HEWH Standard.WattHours (Wh)"=w71) -> (w69:T5)
          }
          frame "D" {
            n14 = Unbundle By Name(w73) -> ("HEWH Specific DAQ.HEWH Data.PRAT.TC4"=w72:dbl, "HEWH Specific DAQ.HEWH Data.PRAT.Power (Watts) D"=w76:dbl, "HEWH Specific DAQ.HEWH Data.PRAT.WattHours (Wh) D"=w75:dbl)
            n15 = Bundle By Name(cluster=w73, "HEWH Specific DAQ.HEWH Data.HEWH Standard.TC Tree (AVG)"=w72, "HEWH Specific DAQ.HEWH Data.HEWH Standard.RTD Out (Deg F)"=w72, "HEWH Specific DAQ.HEWH Data.HEWH Standard.Power (Watts)"=w76, "HEWH Specific DAQ.HEWH Data.HEWH Standard.WattHours (Wh)"=w75) -> (w74:T5)
          }
        }
      }
      frame "HEWH", "HEWH RLT" {
        # "Might need to switch the flow rate control to hot flow rate\nrather then cold flow rate like now"
        # "The intellifaucets are nice...but they occationally loose communication It is more reliable to use valves. Intellifaucts are nice for development. You can use in production....but you might need to fiddle with it more. (Re-zero valves, cycle power to unit, and reset power to PLC\n\nI think the main reason i have issues with the intellifaucet is becasue of the MW100 sending commands. If I could search for a new controller...the issues might go away."
        # "The HEWH and RLT have an intellifaucet. So adjust it."
        n16 = call "HEWH Start PID Conditions.vi"("Error In"=w87, "Elapsed Time (sec)"=w88) -> ("Error Out"=w86:errorcluster, "Disable Temp Adjust?"=w78:bool)  [unwired: 8 in]
        n17 = call "HEWH Adjust Temp Flow.vi"("Core HEWH Data Station A"=w91, "MW100 Input"=w84, "Disable Temp Adjust?"=w78, "MW100 Sema"=w85, "GPM Target"=w92, "error in (no error)"=w86, "Elapsed Time (sec)"=w88, "Temperature"="Temperature", "State"="State", "PID gains (Temp)"="PID gains (Temp)", "Debug"=w93, "Adjust Temp Timer"="Adjust Temp Timer", "Use Fuzzy Logic"="Use Fuzzy Logic") -> ("Core HEWH Data out"=w90:T5, "MW100 Output"=w89:refnum<visa-resource-name>, "Adjusting Temp"=→"Adjusting Temp":bool, "error out"=w94:errorcluster)  [unwired: 3 in]
        n18 = Unbundle By Name(w90) -> ("HEWH Specific DAQ.HEWH Data.HEWH Standard.TC Down"=→"TC Down":dbl, "HEWH Specific DAQ.HEWH Data.HEWH Standard.Flow Rate (GPM)"=→"GPM":dbl, "HEWH Specific DAQ.Flow Valve % Open"=→"Intellifaucet %Open":dbl, "HEWH Specific DAQ.HEWH Data.HEWH Standard.Gallons (Gal)"=→"Gallons":dbl)
      }
    }
    n19 = call "HEWH Check End Conditions.vi"("Core HEWH Data in"=w16, "State"=w32, "Loop Rate"=w24, "Elapsed Time (Sec)"=w31, "Purge Time (Seconds)"="Purge Time (Seconds)", "Emerson Flow Meter Data Input"=w14, "Gallon Target"="Gallon Target", "error in (no error)"=w23, "GPM Target"=w27, "Use Emerson 5700?"=w15, "Pressurization Time (sec)"="Pressurization Time (sec)") -> ("Core HEWH Data out"=w33:T5, "Terminate"=w26:bool, "Time to Draw Water (Seconds)"=→"Time to Draw Water (Seconds)":T2, "error out"=w34:errorcluster)  [unwired: 1 in]
    n20 = call "HEWH 15sec Processing Delay.vi"("Emerson Flow Meter Data Output"=w14, "Elapsed Time (sec)"=w31, "Use Emerson 5700?"=w15, "State"=w32, "error in (no error)"=w34, "Core HEWH Data in"=w33) -> ("error out"=w41:errorcluster, "Core HEWH Data out"=w42:T5)  [unwired: 4 in]
    n21 = call <vilib>:"Clear Errors.vi"("error in (no error)"=w41) -> ("error out"=w43:errorcluster)  [unwired: 5 in, 1 out]
  }
  "error out" <- w10
  "Core HEWH Data out" <- w11
  "MW100 Out" <- w13
